vi "traceW.vi"(11 "x":dbl[][](array[numeric])) -> (3 "ss":dbl)   [LabVIEW 2014]
uses:
  <vilib>/Analysis/baseanly.llb/Real Dot Product.vi
  <vilib>/Analysis/NI_AALBase.lvlib
panel:
  out "SS_OUT":dbl
  out "fac":dbl
  out "p":i32
  out "n":i32
  in  "u":dbl[](array[numeric])
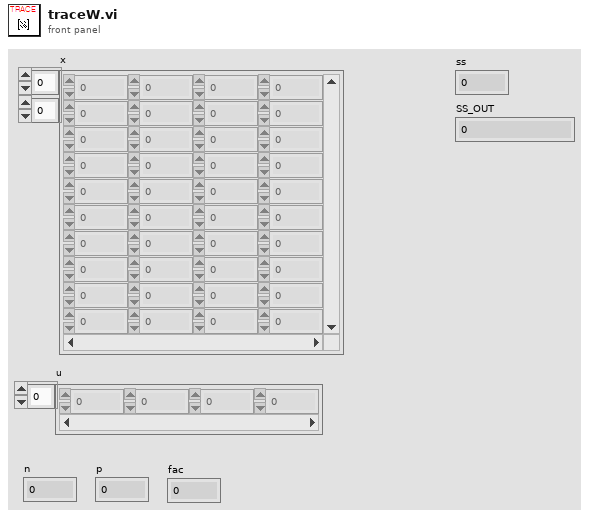
[diagram p1: front panel]
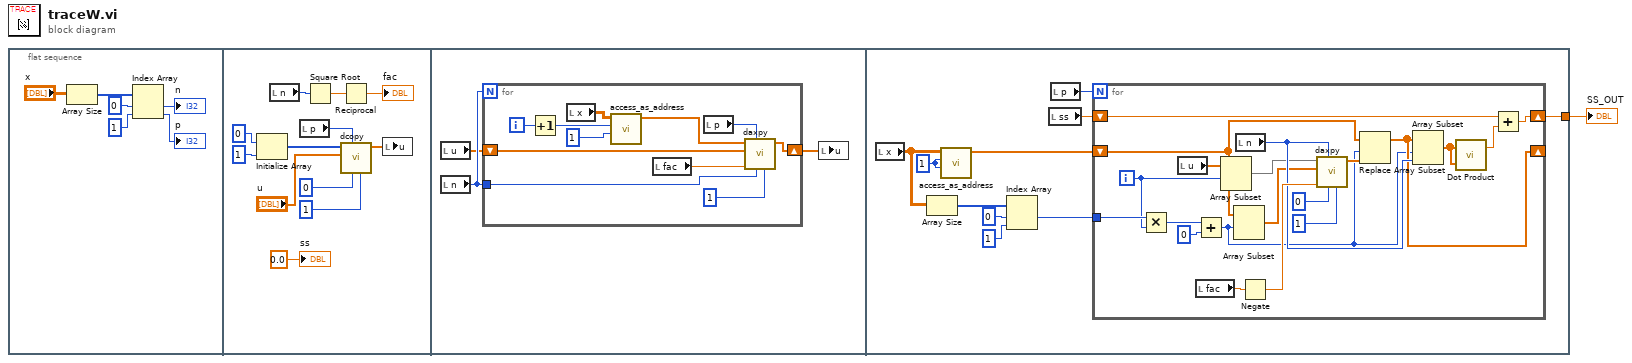
[diagram p0: block diagram]
diagram:
  n1 = flat-sequence {
    tunnel: [w41] -> w1
    frame #0 {
      n2 = Array Size(array="x") -> (size(s)=w6:i32[])
      n3 = Index Array(array=w6, index #1=0 ("index"), index #2=1 ("index")) -> (element #1=→"n":i32, element #2=→"p":i32)
    }
    frame #1 {
      n4 = Initialize Array(0, 1) -> (w18:i32[])
      n5 = local read "n"() -> (w9:i32)
      n6 = local read "p"() -> (w8:i32)
      n7 = Square Root(x=w9) -> (sqrt(x)=w19:dbl)
      n8 = Reciprocal(x=w19) -> (1/x=→"fac":dbl)
      n9 = call "dcopy.vi"("incy"=1 ("incx"), "incx"=0, "n"=w8, "dy"="u", "dx"=w18) -> ("dy_copied"=w12:dbl[])  [unwired: 6 in]
      n10 = local write "u"(w12) -> ()
      "ss" <- 0.0 ("ss")
    }
    frame #2 {
      n11 = local read "u"() -> (w21:dbl[])
      n12 = local read "n"() -> (w22:i32)
      n13 = for {
        N: w22 -> [_]
        tunnel: w22 -> [w32]
        shift-right: [w29] -> w20
        shift-left: w21 -> [w30]
        i -> [w25]
        n14 = Increment(x=w25) -> (x+1=w24:i32)
        n15 = local read "x"() -> (w27:dbl[][])
        n16 = call "access_as_address.vi"("column number"=1, "row number"=w24, "Array"=w27) -> ("subarray"=w26:dbl[])  [unwired: 8 in]
        n17 = local read "fac"() -> (w28:dbl)
        n18 = local read "p"() -> (w33:i32)
        n19 = call "daxpy.vi"("incy"=1, "incx"=w32, "n"=w33, "da"=w28, "dy"=w30, "dx"=w26) -> ("daxpy_result"=w29:dbl[])  [unwired: 5 in]
      }
      n20 = local write "u"(w20) -> ()
    }
    frame #3 {
      w40 = 1 ("row number")
      n21 = local read "x"() -> (w38:dbl[][])
      n22 = Array Size(array=w38) -> (size(s)=w37:i32[])
      n23 = call "access_as_address.vi"("column number"=w40, "row number"=w40, "Array"=w38) -> ("subarray"=w39:dbl[])  [unwired: 8 in]
      n24 = Index Array(array=w37, index #1=0 ("index"), index #2=1 ("index")) -> (element #1=w34:i32)  [unwired: 1 out]
      n25 = local read "ss"() -> (w42:dbl)
      n26 = local read "p"() -> (w43:i32)
      n27 = for {
        N: w43 -> [_]
        shift-right: [w46] -> _
        shift-left: w39 -> [w54]
        shift-right: [w56] -> w41
        shift-left: w42 -> [w55]
        tunnel: w34 -> [w49]
        i -> [w47]
        n28 = Multiply(x=w49, y=w47) -> (x*y=w48:i32)
        n29 = local read "u"() -> (w63:dbl[])
        n30 = Add(x=w48, y=0) -> (x+y=w44:i32)
        n31 = local read "fac"() -> (w62:dbl)
        n32 = Array Subset(array=w63, index=w47) -> (w50:dbl[])  [unwired: 1 in]
        n33 = Array Subset(array=w54, index=w44) -> (w51:dbl[])  [unwired: 1 in]
        n34 = local read "n"() -> (w53:i32)
        n35 = Negate(x=w62) -> (-x=w61:dbl)
        n36 = call "daxpy.vi"("incy"=1, "incx"=0, "n"=w53, "da"=w61, "dy"=w51, "dx"=w50) -> ("daxpy_result"=w58:dbl[])  [unwired: 5 in]
        n37 = Replace Array Subset(array=w54, new element=w58, index=w44) -> (w46:dbl[])
        n38 = Array Subset(array=w46, index=w44, length=w53) -> (w52:dbl[])
        n39 = call-poly <vilib>:"Dot Product.vi"("Y Vector"=w52, "X Vector"=w52) -> ("X * Y"=w57:dbl)  [unwired: 1 out]
        n40 = Add(x=w55, y=w57) -> (x+y=w56:dbl)
      }
    }
  }
  "SS_OUT" <- w1
